vi "TickCtl (SubVI).vi"(8 "error in (no error)":errorcluster, 10 "GUI_TickCtl":refnum<vi>[](array[refnum]), 11 "TblParam":sgl[](array[numeric])) -> (0 "error out":errorcluster)   [LabVIEW 2017]
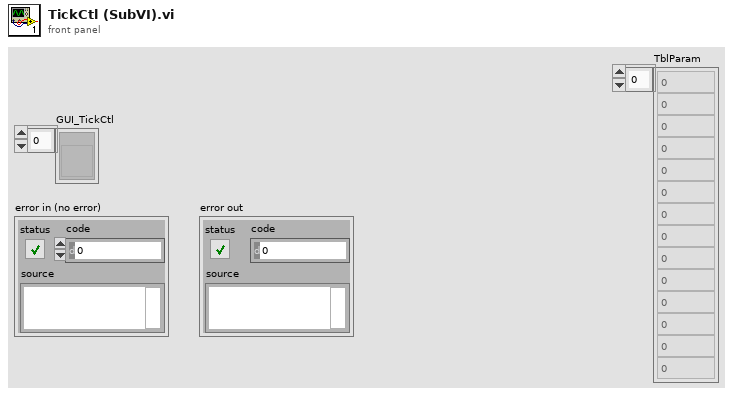
[diagram p1: front panel]
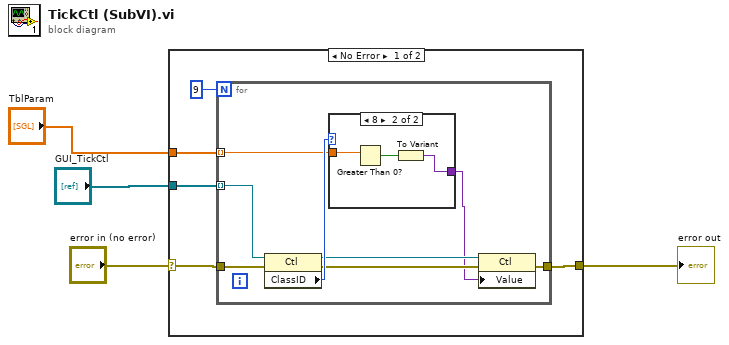
[diagram p0: block diagram]
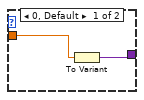
[diagram p2: hidden frame]
diagram:
  n1 = case shown="No Error" "error in (no error)" {
    selector: "error in (no error)" -> [w7 w23]
    tunnel: "TblParam" -> [w9 _]
    tunnel: "GUI_TickCtl" -> [w8 _]
    tunnel: [w6 w23] -> w4
    frame No Error {
      n2 = for {
        N: 9 -> [_]
        tunnel: w8 -> [w15] mode=indexing
        tunnel: w9 -> [w16] mode=indexing
        tunnel: w7 -> [w12]
        tunnel: [w11] -> w6
        n3 = property class="Ctl"(reference=w15, error in=w12) -> (reference out=w14:refnum<vi>, error out=w13:errorcluster, "ClassID"=w17:u32)
        n4 = case shown="8" w17 {
          tunnel: w16 -> [w18 w21]
          tunnel: [w19 w22] -> w10
          frame 0, Default {
            n5 = To Variant(anything=w18) -> (Variant=w19:variant)
          }
          frame 8 {
            n6 = Greater Than 0?(x=w21) -> (x > 0?=w20:bool)
            n7 = To Variant(anything=w20) -> (Variant=w22:variant)
          }
        }
        n8 = property class="Ctl"(reference=w14, error in=w13, "Value"=w10) -> (error out=w11:errorcluster)  [unwired: 1 out]
      }
    }
    frame Error {
    }
  }
  "error out" <- w4
